vi "PMT-lock-in ROTATION -single rotation-withplot.vi"(0 "Time":dbl=2000.0, 1 "start":dbl=-0.2, 4 "stop":dbl=0.4, 5 "error in":errorcluster, 6 "Frequency (Hz)":dbl=2000.0, 7 "velocity (mm/s)":dbl=0.01, 11 "APD counter source":tag="/Dev1/PFI0", 12 "Interval (ms)":dbl=100.0) -> (19 "error out":errorcluster)   [LabVIEW 2010]
uses:
  <vilib>/DAQmx/read.llb/DAQmx Read (Counter 1D U32 1Chan NSamp).vi
  <vilib>/DAQmx/read.llb/DAQmx Read (Analog 1D DBL NChan 1Samp).vi
  <vilib>/DAQmx/create/channels.llb/DAQmx Create Channel (AI-Voltage-Basic).vi
  <vilib>/DAQmx/configure/timing.llb/DAQmx Timing (Sample Clock).vi
  <vilib>/DAQmx/create/channels.llb/DAQmx Create Channel (CI-Semi Period).vi
  <vilib>/DAQmx/configure/timing.llb/DAQmx Timing (Implicit).vi
  <vilib>/daqmx/miscellaneous.llb/DAQmx Fill In Error Info.vi
  <vilib>/Utility/file.llb/Write To Spreadsheet File (DBL).vi
  Program Files/National Instruments/LabVIEW 2010/resource/objmgr/daqmx.rc
  <userlib>/Newport ESP301/Newport ESP301.lvlib
  <vilib>/Analysis/NI_AALBase.lvlib
panel:
  out "Numeric":dbl
  out "XY Graph 4":cluster{dbl[], dbl[]}(graph)
  in  "Interval":dbl
  in  "Stop":dbl
  in  "Start":dbl
  in  "MG17Motor":refnum<k7>(container)
  out "Y":cdb[](array[numeric])
  out "lock-in":cdb[](array[numeric])
  in  "Photodiode lock-in":tag="Dev1/ai1:2"
  out "Lock-in ave":cdb[](array[numeric])=[1575.618405636581-1354.780267530867i, 2376.9087046503932-757.7461705623398i, 430.26344393445436-2001.7808909348576i, 274.00880357824946-3233.9431935405287i, 888.5075748796727-579.8898083376234i, -1288.5272699325-2538.9581308616175i, 1814.519128631189-3653.715758651259i, 2580.0434389062198-2021.0268672269435i, -866.6428201396346+76.21564286365829i, 1521.4600711033984-2572.1678721325943i, -595.4162527325557-2083.0235307435746i, -2213.651439951863-2304.726379582989i, -1581.3102291517034-3444.508965588943i, 2963.698823411756-3466.251761677201i, 481.31874465992325-2590.4156650248883i, 1077.5453470367086-2271.1674251376476i, 198.06969556939967-3519.1421862721854i, 2126.002010792124-1554.2537826475386i, 1951.9736792597407-5745.697506603049i, -1202.1061809811476-5047.9372242667605i, -1253.5217513533728-1443.9298926030515i, -2137.041153840351-4836.853717701188i, 2212.4903951925257-1208.6810705385744i, 1183.0549708527803-3817.098140391271i, 2431.6697161632046-2314.138255588717i, -502.1017800179644-3590.6658275236773i, 1823.0672697368907-2486.578868433814i, 325.79092146215373-3610.284263297886i, 569.0882415193973-1599.4282971963353i, 3604.4445594698154-4299.084099003819i, -1486.317634221812-3764.9834009605543i, -936.0268941833114-1644.1672785866663i, 292.4719293881775-2213.542158236794i, 318.9126890705529-3399.5505121690685i, 2176.4211819849957-1734.6139938020951i, -953.3489073228936-1819.9444385577192i, 2588.5498347626085-1667.03179470835i, -1029.7581374768777-4091.2934217259995i, 2021.0392661929118-2696.896974507213i, 1446.7594755721875-3062.0656501211965i, 896.0183055508568-3577.8143635934734i, 500.62347573888036-4189.918427475723i, 110.42931799715957-3202.0014798287652i, 1380.892527892701-31.67874295288169i, 2004.357779053466-3723.2441111391868i, 1533.3345211084109-5425.565755113332i, 4364.135929502945-2877.434664532994i, 1257.8199986491823-5604.62816893496i, 1255.4653962401853-3212.376740460875i, 1308.1516341284914-1771.8716117456422i, 5153.052050385331-2811.678589495896i, 1355.9361808963736-3679.095640287204i, 2468.122406976211-64.5200597946781i, -191.8770322387612-3987.068653237768i, 2216.7815087525064-3974.7865562586812i, 811.1736358070949-2695.2342284855467i, 2799.6354672167445-377.1654452867725i, 1232.1759963228278-2564.1871307341107i, -612.1595688464043-795.2702470245148i, 1491.1312054147534-2415.392098859457i, 2503.052266186264-2070.3324822117393i, 1232.7885043542053-4349.227949033147i, 2198.166504463149-3917.0252303013986i, 3670.498177889123-4750.584371253087i, 1049.7577709417797-4272.772555595173i, 5219.707004524125-1875.1488939589096i, 1775.370073504267-1636.5169106622857i, 182.0049681671236-4800.672748236866i, 1484.4660201569386-2355.873769649259i, 1180.3743379538816-3096.2588923411595i, 772.839482950376-1303.4236258336866i, 1549.9878546671623-6153.910783877218i, 47.914672339113324-2471.481982105196i, -2996.873617434996-4030.907310697404i, 2179.4047715196602-2190.9435841994223i, -1253.917311902031-4251.133411229375i, -666.0664524021325-2716.4388438333253i, 2366.5511527892622-4388.085109381615i, 1144.487614423424-3108.4279901249i, 3215.2297186251376-3286.077498973359i, -2099.4212370216474-3992.9683286935906i, 821.6004184060433-3180.0929231557093i, 505.29024588883806-1175.490759941422i, 459.6869492084121-5440.359151670178i, 897.1741551100467-2797.6567465972225i, -715.251854275629-4444.1499126874505i, -392.6708280128788-4277.723316797537i, 1818.1920888630784-2260.469810578464i, 2820.4585961324674-3295.0628100957574i, 901.7716895731513-3808.91683958497i, 2197.026105691963-1790.338710230202i, 3516.3398245212875-4396.432964245725i, 3140.9683427347954-3560.206476639805i, -297.4601035595252-6652.839678247998i, 2423.649156341772-3610.5951839245477i, -669.3988195260619-5549.785379880692i, 2140.7327741099975-1863.2281007983468i, 1183.481250478131-5805.0618816517135i, 649.705046261852-4561.171961145662i, 536.6278860470271-6367.077600133586i, 2950.853999097596-4102.535083107555i, 2600.519648862765-2214.5762658985313i, 2377.7508979599465-5388.334575899893i, 1808.695648329345-4369.762899527957i, -1374.0277904112904-1593.153029070302i, 1091.7884376939294-1260.670032252601i, 304.1154584761832-5567.168439100472i, -981.4392899572041-5080.2068823010795i, 2334.8207050837145-5195.204705625067i, 1026.0461525520295-2069.3530721213815i, 2451.6963287267326-5204.362144252449i, -457.07442892523954-4530.848217232627i, 1448.4675260975769-3703.542478400782i, -139.3301300114125-6171.845273134681i, -638.5494225411103-3042.7814299211786i, 836.4493886595066-5194.499239015591i, 4083.2545653137086-3715.3991686367217i, 2810.0108324746325-2942.6225697417813i, 759.4212715648375-2377.1759813419703i, 2381.5026388043298-5282.685521239267i, 3842.3491663279096-3538.1939118229166i, 4107.981184439802-4482.028922780051i, 4188.535704530702-4431.638680818972i, 2622.805061687113-3225.044270443636i, 2320.0408164989244-5506.118437667573i, 4733.871150582911-6726.079493601502i, 1215.8496144855626-2012.8662115061009i, -533.2529951016124-3411.0893784284817i, 3644.173088205299-3633.0667675324107i, 3270.672994482886-3873.4145432672726i, 2111.2936695423305-3534.34925451735i, 2154.2353903099734-2399.833843699712i, 5054.243227569061-2753.803721852707i, -56.45164399137748-4038.4049421212617i, 1478.965032062944-8093.284127952804i, 2387.809869177338-3421.6143761555795i, 905.8600180472704-4280.089794207029i, 1167.9761571101933-4807.61154339191i, 2615.006809102998-5061.344202856609i, 5736.0218405457545-7406.057718262208i, 2087.149131407617-1955.3279233788548i, 948.4800480918925-4594.139729285302i, 3139.012629546095-6765.397296171153i, 1420.470992347951-5382.169689346777i, 3445.7663547749776-4544.194313423124i, 3201.513005693168-2941.5999006229986i, 3049.9336370159685-1158.007902042452i, 2861.5908669288833-5042.927937990892i, 3095.9352635655273-9215.194383301981i, 2039.8615756080867-3732.315434450052i, 1403.8112843594183-1596.2751532830828i, 2545.8562757136283-5314.4090804453945i, 1215.3340538700709-2860.4819306523045i, 511.8716581082042-6949.692527491928i, 1809.8402634609465-4170.701581866224i, 1983.4607774157303-6035.908248310845i, 2752.5388621309908-6089.687105796719i, 369.47893038169406-5111.808157222528i, 3094.2046544310415-6055.085104732612i, 393.2964691176897-6516.055517047396i, 2888.0442175269045-7598.7063277771795i, 2031.1829482164803-4507.499609177696i, 1286.689454116021-6167.992540949457i, 5898.792902286471-6307.398221312562i, -752.3240471967462-7036.154374283361i, 661.7732013776628-9053.440012958048i, 1343.9313451110952-7300.1365150680385i, 1409.2166078499054-4353.6006586350695i, 1319.979807062355-6098.946164044407i, 2650.6676320636348-6713.891596934963i, 674.1552177359422-5915.62441705174i, 3774.0240383235837-6240.564229457563i, 2442.2611560948644-6293.2324371160375i, 3195.663634320999-6960.896051196942i, -1440.7125037445865-5874.2812237151875i, 2556.676353026318-2669.1223205575393i, -177.91447697888032-4420.9979098207i, 918.2672041740103-2696.085793660552i, 266.11624646743354-7089.299508598139i, 465.92571257727855-3112.388597098675i, 2682.0623447087337-7824.876084863631i, 4426.760086777614-7163.480624926065i, 72.418199475638-5525.248134633922i, 2840.4684511518744-4430.394194406008i, 2819.18026213846-4090.997860405245i, 3891.8677914991113-5735.681669839178i, 2582.946348733788-6972.788033682008i, 4396.446981258371-5272.910199984774i, 2527.0694028279963-7180.483205691042i, 2005.8355590023666-5022.379414766889i, 4150.5132191837665-7929.531405210346i, 1302.0321986691608-6354.158853952622i, 3276.071312110827-7137.673634990922i, 4112.351344872533-6809.4887694552235i, 3233.240880674217-5713.885210511878i, 2294.125519119039-7149.913211378586i, 2521.825788957482-5327.505448819114i, 4472.642628671886-6719.528858266076i, 1156.570051540259-6042.931068163441i, 4263.312379237701-7354.80045290692i, 3231.5904372730024-8603.646792538973i, 2954.9382594092604-10493.056880345923i, 1386.493795027244-4351.668054824362i, 3225.5987563761487-7125.386281538512i, 2998.2482884144883-8640.063883320861i, 5034.563279599767-6334.290206381059i, 5415.675544216023-7053.302845855882i, 5696.215560860752-4634.538974053647i, 3641.080159251063-6410.635909506378i, 3047.4325898702286-6570.782759795123i, 3335.9774335594325-7959.350599243415i, 1034.8217959811998-9471.783462254887i, 4472.18270995681-7972.728001848677i, 1687.1669694183852-7691.372201957279i, 3838.7682454706164-4608.7353483079205i, 2789.723450221373-6735.727257013259i, -100.86652927079496-8280.414793254728i, 2691.163672840396-8195.965205608558i, 3135.3844380749388-4334.554385434998i, 4754.501592156671-8150.319779417582i, 3152.46020482383-5267.56497828292i, 3345.6422634325527-7666.082415105115i, 4268.253179283182-6228.07112408391i, 2468.284969279949-7082.494872178709i, 5146.391606558882-9442.984964408635i, 3017.350279911123-6366.988520079154i, 2983.935453577272-8328.674529063186i, 1779.3304772234042-5359.456608012244i, 3510.110664729989-7196.888677953726i, 2937.7827141235925-7916.234771289581i, 3390.6936769238473-6158.017390219011i, 5116.173881936087-8156.452921998013i, 4815.733340806664-7292.728942666812i, 4745.333271691776-8481.200756112174i, 5365.885743637579-4990.0099400448125i, 4782.323630181974-8164.634702569512i, 3551.0138437730548-10338.68778651241i, 4487.380002158204-8108.007387676075i, 3286.690337470376-7921.318236867741i, 3376.0031275370734-7442.806636330388i, 2265.3725204363504-8070.769839902126i, 807.157044198946-8219.94254152485i, 2523.9981278773407-7171.667112435127i, 3364.1321813453346-7864.664176825664i, 2853.3817229355914-9339.871887243396i, 6505.60918603455-8014.805912068681i, 4548.785193789941-7068.753744337186i, 6491.907317829052-11153.440489008437i, 4119.273108721625-11156.272587046135i, 4468.012071037022-7603.962904432309i, 2445.5704319838724-6135.840418565561i, 5415.917334042106-7934.862125438665i, 4375.69619385447-10252.680472604265i, 3300.624533464226-8981.870565534917i, 6416.737775940689-8055.459849998011i, 2147.0423638877305-7800.421166609077i, 3470.9244469034734-9652.502973243401i, 3834.944754020379-8997.730145163221i, 5191.853577022501-7983.604511323078i, 6926.471309680483-9982.320605300636i, 5565.609902585673-8801.550363525452i, 4425.618931406877-9686.465846148525i, 4750.691251487348-7229.1346402430445i, 6060.328452057632-8410.696096223492i, 8642.740346806098-10615.813484936069i, 4000.851811107144-7713.603497846788i, 5340.429627507394-5564.470385899507i, 4246.436081468988-8451.254786399202i, 5142.1808707504315-8970.507919104013i, 5849.381578431081-10722.75061539895i, 4743.6306751765815-10982.737699019313i, 3662.8719327485355-9718.164212385662i, 6375.327301060715-12608.26617199092i, 3208.3276860287815-13184.554856913566i, 6462.5111596734905-13846.584482642662i, 6450.4053011412-13032.71550445879i, 6611.623790823844-12964.883545718125i, 3012.9070584814795-12009.812713614641i, 8276.19374857804-9520.97744420273i, 6088.451995458484-12662.88351339309i, 7433.678429940602-12919.825710196095i, 2852.2427242612903-12793.526883177705i, 4723.55739094081-11279.148288208788i, 3539.2212584925037-12636.463067970388i, 3127.94039402949-13919.258461339436i, 4042.7498170819094-10438.47267823518i, 3313.8462354475123-10185.0005143772i, 2083.0105152702654-13337.796688349425i, 4415.742453714986-12296.444745051213i, 2333.6873585833296-12599.213531007452i, 6541.907912842064-16769.193637528468i, 3868.710658608924-12774.742387506203i, 3516.06243618668-13159.889412777684i, 3703.0889476515376-13765.671181982048i, 3675.6227579825686-14310.612784302477i, 3812.441605180332-10887.472287294133i, 1397.0828808435276-13734.236307413365i, 3938.7295726058055-14035.867119071843i, 1825.260919517559-15010.104724879697i, 3484.4101933582256-13615.583679334506i, 6045.007586638047-14483.223663464456i, 2266.133309683563-12932.45957066616i, 1216.366596052904-12096.177750738301i, 3094.775105021804-13466.285271132703i, 1343.0682931154638-15830.12324274869i, 3723.6282011488-12088.74110571i, 527.3450422106561-14712.257687544445i, 3319.7368165379435-11364.549104548822i, 2297.976854474832-14017.971969481849i, 848.5790411140356-13690.064307972925i, 2033.8439056264206-11773.725311700986i, 770.4447513128919-15217.642846257875i, 1853.0905652266492-14177.448493715083i, 1792.8092173986097-14424.43565501314i, 1207.0272513039884-11125.9188243898i, 984.5665559117601-10123.787770201357i, 1934.1627600043782-13763.568829080928i, 3319.8803814773346-12100.916557943508i, -682.4754463650166-12295.072338224982i, 1010.1082259658396-12544.228333526644i, 1443.8085907844304-8732.055376323178i, 822.8876816006555-9900.247376109055i, 1611.2724688688406-10996.094241351546i, 1446.180298133071-9565.616335014467i, 939.6520132331581-10622.586263289028i, 642.985545092809-14054.122868742952i, -1312.8387064380534-7879.215014987034i, -422.0499978802597-8294.918016716652i, 945.0198134398789-8873.172496645318i, -1874.029242704319-7324.3221632276i, -911.5088864967161-6727.6651678308735i, -814.0487519371331-7309.334312834168i, -8.383164099631617-7717.6915717605325i, 1244.481834156355-6580.924107883921i, 2358.0710913512617-5494.890411171763i, 715.2405105254029-4605.4887026423075i, -1350.4053391373088-6162.0264940668i, 840.2512985319834-4720.024981664563i, 244.63112371075078-5910.131730889196i, -503.3729172442221-4348.932318470168i, 815.7115745334273-4384.529220903181i, -443.19112139589043-4965.184510612029i, 210.21261276302315-3120.9557463527262i, -1835.4249558866986-2538.6010144168818i, -1123.917602737967-3779.9767572298338i, 660.1740596516721-1772.286398958819i, 1102.1856160660475-964.6607531448776i, -733.3571432042307-5349.184027686582i, 839.6615019045682-3137.2615174093594i, -1871.8261810359465-1294.6855534867075i, 1531.2808862634479-1171.163074759485i, 667.9924422761186-2953.8871853082583i, 129.02940560864587-189.19271316344606i, 3182.1888736477886-2735.789162005561i, 1168.9250333431555-272.33635084978556i, -1123.7362237647644-3604.17838791847i, -1395.1851983393085-1895.665289942973i, -571.7555591978203+1071.1038162245345i, -2170.2022145503834-3487.684684038925i, -776.6818955944391-480.1729930056903i, -1854.886019995663-800.1289791333481i, -1176.1015445632427-1424.3339818833902i, 1687.3748265199076-2187.0524559081196i]
  out "Signal ave":cdb[](array[numeric])=[19973.709551616634+2137.68316236515i, 17641.679526528722-590.6971995647476i, 18964.42920598725+784.4848963807648i, 20443.339940618058-1292.7777293085899i, 18783.5054836337-586.7016703281453i, 17591.273408972083+346.8128608267923i, 14435.708762127228+355.6367697407369i, 17955.809692629875+970.7427647798825i, 18901.743132287455+2350.1528064430026i, 16181.835360198562+769.9403678944353i, 18619.57566660758+101.29369171834527i, 19714.78151159957+2874.616325663279i, 19910.019889764048+1971.0987272756875i, 18778.497214983232+2012.7224915615561i, 19243.150553663443-879.2727034505004i, 18798.14167792132+939.01546450782i, 22779.513628065473+2910.1695280022336i, 21017.14310563447+1146.5352790872914i, 22370.876093470342+3759.021856982118i, 22038.151641544195+2119.3106285164895i, 20021.386988714767+1152.1162632125843i, 21872.217528511355+2454.1895448417736i, 21877.851134885925-117.33523182960502i, 21685.988414070882+4080.139956736632i, 21687.794636398055+4650.407322525038i, 23216.427067114826+365.3502429257846i, 18649.66991238834+3200.034227192907i, 20283.547667981533+121.5380892072013i, 21996.53785526474+1247.1035231835428i, 23187.751052088097+1585.2474258033446i, 25751.290144574323+768.5946057235767i, 23093.45018600484+2197.702088670342i, 21645.07391481427-149.9515993110738i, 17628.63439529744+3672.495048304777i, 19950.242163716157+2209.1177096797396i, 20492.098732128667+1793.4072912054614i, 19449.224016281816+3379.3313636089556i, 20175.360044553425+3508.299044497772i, 21079.557314354697+1546.639742437651i, 22785.549397207353-591.3827688982097i, 22077.17826531066+3270.940314774405i, 23398.14028789829+2830.2652332386506i, 20646.262168996647-126.72623217786679i, 22349.320346499582-31.902379363178866i, 24243.400587859025+3426.5148490693373i, 21916.085290303516+2529.5297370956946i, 21981.748030513918+1530.0184869116495i, 22220.24447104533+2731.5080444137875i, 22945.91165334838+1386.5913250565343i, 22707.88746616709+959.3818222670607i, 20273.53720619981-63.13732196241676i, 22042.231102113492-19.60268674334982i, 25650.121706604354-1289.452205628714i, 22690.294811693293+1628.8665056493544i, 23952.7408549437+1505.7600996787273i, 22845.286418081443+855.7065280668362i, 24593.853888002035-55.12625244238829i, 25077.041608896685+1491.9633380572377i, 25068.358254862625+1317.2389077564858i, 23548.43171700486+1611.2100374579366i, 25969.705099151113+388.3654069151239i, 23702.173502861428+2015.8803757325109i, 25965.49633041593+2170.8831987562753i, 26701.80741871982+278.2637036757209i, 26860.199652986015-3275.5802176156444i, 26488.641761538747+1822.8973333641702i, 24914.763925257383-1756.5451070743327i, 24540.892320736584+2643.699533046424i, 26346.68660390194+2976.8179266998004i, 23236.44710958339-456.99626328409965i, 25552.947774671287+2296.2714910902637i, 24809.85032506418+3461.188281980759i, 27374.123718323208+2344.9869732905986i, 26281.683954696782+3069.656547340776i, 26683.785078787205+713.8589978246326i, 27018.240909618165+1228.2539625246457i, 26299.67568231255+2257.2555548593223i, 24921.943873921533+3476.991048682698i, 27963.693598569236+2024.1104863223575i, 25338.366480063796+1460.8181084882951i, 29096.956578838577+2852.7644971285185i, 29099.59494568991+2708.1173513220506i, 27156.515231099107+1477.3327428415637i, 27621.35094330793+254.29043438568937i, 25450.491878025037+2740.910850675434i, 26928.105928600937+309.4305324651831i, 27887.833450880145+245.37632737638654i, 25628.298853828666-991.6321417652896i, 29018.592445695496+4265.022956712465i, 27655.547923423754+3309.082973772353i, 27654.10848220132+503.6750065510531i, 28091.70288293553+3312.482883066248i, 28857.703507639355+2717.4979820902295i, 29239.16353925298+846.9422025653236i, 27633.945284273672+950.8074087747111i, 30817.8953983305+183.09505881489707i, 28716.053737316877+1359.63211416521i, 31368.296864577864+1285.0617682950906i, 30394.766926577733-64.2060995609443i, 30639.02392489712+1903.0823876456561i, 29889.982496973058+1288.5353310469095i, 30092.068332835745+2556.940302097282i, 28447.660023560045+131.4721229425815i, 33747.72123923668+2604.592206852926i, 30733.81223686092+1711.5814227720543i, 32109.547759341844+1571.950999302157i, 32242.31561562917+1393.6930049698697i, 32590.39968579184+994.9027982538349i, 30826.777950969077+4965.444045031032i, 32436.07511683829-508.22337870489105i, 31859.064193175956+335.5035319454363i, 30734.76537878668+2275.0504484911216i, 31616.526804989484+1156.3420961595307i, 31726.168231515585+2058.313894580561i, 34072.22274345362+1727.996383661928i, 30735.246560596046+607.2659759455697i, 32722.61019328942-304.4169498497065i, 33379.36582025203+1398.4899414019935i, 31283.35823156214+2067.1972169709866i, 34276.5412407718+1801.202047655149i, 32524.364278892383+411.72304514708674i, 32911.84465016063+3106.4363661109296i, 34144.52154366048-674.2921396242247i, 32213.46494533557+1497.193235188105i, 33359.57364425402+4890.421863521732i, 33020.841577154395+2432.091933361664i, 34645.64981776737+992.224198121691i, 34935.86915287571+3139.85366888939i, 34053.63229435785+1902.4338552972958i, 35190.1445344589+3684.5700980275315i, 33810.07920022588+1946.6764540660133i, 37192.40763536752+2291.5382514440716i, 34390.850778472406+3552.7818186234745i, 36523.90485411221+3552.3812997237105i, 35928.96030095971+1527.1878693068945i, 35101.623255081235-422.12491807187314i, 35874.32004068537+3995.9013181685286i, 38245.00604558553+2794.963564772352i, 36282.57405831285+2289.9622033544665i, 35801.267580883265+4612.021916772325i, 37913.50698705951+1810.1753523431848i, 37868.538496427704+1191.0366636643264i, 35433.08521708961+3281.138887103279i, 39933.430938674246+907.6894155147743i, 37197.9365283357+473.98998197129714i, 36551.44941131433+334.6769403013012i, 37718.6079672964+405.8678874777269i, 35936.98611716157+3673.2883676638235i, 37899.705096743186+4498.070132155895i, 39012.34346929452+3905.593779920433i, 38502.32920850229+2135.9721312509164i, 40447.2529957549+1518.378412117692i, 40209.58476152285+3464.9226117868006i, 39179.87322920747+4498.566856320326i, 40135.85181622762+1967.805904084847i, 39633.94042233719+4445.4072774265205i, 41424.06052762676+2912.18379277977i, 40531.01365901944+3373.1736448150123i, 38643.12888467001+4193.790711494204i, 39027.153852419324+2248.685628882114i, 44654.11961569351+952.1317955274311i, 39944.82064738734+1383.9756797142338i, 42636.26359705652+1343.2573124938638i, 43028.84813983183+3538.8834076296994i, 40359.93711784901+4334.420837491159i, 38658.037995574734+2261.4151424959105i, 38420.68131891876+1264.5325731248104i, 43911.426293769684+747.554605029913i, 38009.551880513834+3552.0732622099863i, 44022.31679663538+2495.6957059671213i, 44496.056984881165+1604.7394074286194i, 43178.600994714994+2885.0449554090123i, 44198.01437631617+502.34729455858894i, 42764.84151033523+3212.966631358569i, 42592.107908395585+1668.6815654216025i, 46034.78812228002+4455.730401066182i, 46580.98252889817+3778.266571802271i, 42050.55243452278+3758.9881368248584i, 48205.45224925414+3462.2732552830926i, 45118.651222056615+2929.6518139001864i, 46956.83137800294+3894.477330360894i, 45501.89150707532+410.8961765597546i, 47780.722456232+3260.665707046737i, 44659.73126251827+3019.103741251046i, 46104.95132677405+2834.695923843316i, 47438.76549627922+3901.244860974728i, 47574.23814215162+2564.47225164935i, 47333.77920621191+4833.004044079297i, 48674.36715884112+898.7979723580138i, 47913.71587388793+5753.460649058702i, 46680.79468934667+1828.8276025492314i, 48747.78242159783+3830.9906332830196i, 49493.82194100686-1147.7435192922012i, 49238.97020889669+1217.3806166213337i, 49659.41497869748+2896.0220275089414i, 49922.467736578175+976.3014341831184i, 48122.218330009746+4044.246307736089i, 50728.933260013655+2301.9555702623406i, 50426.48650279836+2622.593932015488i, 53111.54386920386+2592.047770207518i, 50379.18284070535+3996.648332231636i, 50833.74129682521+3827.5323787287493i, 50276.528475600244-397.24418561847347i, 52521.73784220521+1215.93732991796i, 50727.59448501055+1587.0299271466995i, 52774.08272609958+3168.678810043082i, 53530.35354307037+3153.616420441528i, 49400.85628930751+2483.4779682878993i, 54576.30053668804+4515.088010859563i, 53210.843520241506+3485.18810442704i, 54808.731176971865+2805.6714446276737i, 54131.65617607714+4708.274692447471i, 52050.97491552243+860.6104775218644i, 53846.03228996166+3144.825781282068i, 56437.45630070019+3781.521907374692i, 56872.44923672083+4740.357738623805i, 56506.976569706574+3571.6972230511424i, 56122.1625694851+5064.461210812666i, 55552.439949603744+3217.5911785784383i, 54197.08525324574+3065.799700794284i, 55351.29814379563+5277.107333139463i, 57022.28910243668+2020.5423545949095i, 57966.34735640804+3790.530471207716i, 59215.871189722464+5746.952903378195i, 55853.27951363862+3370.432688647369i, 57971.10026426304+3902.920247338582i, 55575.962320089995+3946.349866444711i, 53919.41630411781+4190.446809659357i, 55992.59602380357+2597.1179953191076i, 58925.31937109892+1881.3178312811253i, 55152.48768021333+4823.910074913119i, 61550.851147975074+2923.6268947041003i, 58025.31157427309+4423.737991353994i, 59953.05368253878+2628.9658176630023i, 56731.86829871749+2344.614900096433i, 58329.518773108626+4631.775781435258i, 61422.440267130434+2258.5760540698116i, 62045.67950061424+542.0322484292351i, 58957.44508030157+2376.8826163311924i, 59829.80588693156+4530.9213058834985i, 60115.67891516981+7080.701980317283i, 60865.784617930076-392.0492100132247i, 61520.315840997515+1346.916327792884i, 62669.975399233976+920.6776954421268i, 62599.45803377901+4176.317544211401i, 64096.245997110505+4132.454017068202i, 64924.98977651045+3982.623708867158i, 67352.74184301558+3867.9328257361894i, 65408.89287634846+3280.8053428012463i, 64561.08345370794+3457.3649032173084i, 67933.9733797803+4312.1263237779i, 64997.73200022106+5700.128391838776i, 65178.453628589734+5928.007376987131i, 67058.91471038818+4137.3498495279155i, 66422.00948928189+3550.307954967456i, 65439.604361950536+5442.195117047383i, 69707.11726364907+5908.003955378939i, 70501.48114958392+4270.954851555873i, 68099.18287494844+5085.339780590591i, 71207.08603062917+4988.153126414789i, 71305.2745976459+2449.914709389416i, 73299.78008493187+4072.663481611199i, 71198.5333353847+2663.292271019781i, 72747.37634043346+2066.3868712407207i, 72537.35439987564+5332.394637655405i, 72822.80196767036+4717.687067031672i, 74110.37560523134+4070.0717297584083i, 74090.76916031171+3712.8083610513972i, 77532.49749680342+3916.912486215792i, 77855.61000565469+4244.644783549382i, 80141.13389083299+3568.9960639135816i, 80096.29528802745+4478.341703421639i, 78878.80665780169+5271.018286940097i, 80834.22339497734+6058.2314951689605i, 82551.58375247684+2968.2393827156966i, 79961.11900757885+4036.8180392654126i, 85322.05433041895+4375.581534713559i, 85674.32244881566+4120.994111269414i, 85814.23398049959+2778.1549316530813i, 87229.4987262963+3301.127968348004i, 89089.2304542043+6634.044264508146i, 90207.16067887297+5700.129391349136i, 92896.56488139722+3753.9567239860407i, 93358.11169050074+5741.308700361177i, 92862.62270723494+7308.441357457153i, 94044.8749091163+5317.911739504252i, 97206.05897811196+7493.372092573997i, 95203.60075421458+6466.563427418022i, 96635.2218642239+6360.661086563576i, 99223.00304946786+5944.922717782365i, 99604.33261943738+8341.485217075271i, 99205.87135539162+4700.30084507866i, 99636.59329708801+5280.88441507546i, 100305.18791388128+7899.87619089107i, 102050.84518525499+7039.313760840313i, 101963.09211888627+4196.707865676357i, 104815.58839322721+4291.404572448898i, 106007.31466316282+6235.22732367124i, 106609.44430278087+5759.485308884078i, 103894.51820826704+6253.566531548679i, 104537.244768498+4935.355572246167i, 104494.31290463262+9238.708466288446i, 104556.61686128186+7305.011221231405i, 103116.14370030162+8340.001515539703i, 101531.33165206132+6108.114347233464i, 104220.65301927809+8029.629028542398i, 102930.77897828724+6102.658516566913i, 102006.32555247868+6686.477306991325i, 101456.17809984833+7585.061130233768i, 101487.76699549012+9933.727119501966i, 99739.96200283422+7162.085932781197i, 96871.99872036949+6277.45473389155i, 98567.49091580088+7496.920314989954i, 96082.9326907551+5292.609874919571i, 92739.44655875764+4948.650055115154i, 91871.171097579+8349.247350111758i, 91843.8898712052+6009.600483014275i, 89160.6478151269+4589.728818531861i, 85472.86835798915+7151.307495948784i, 84104.77649438687+5867.1315478274355i, 79616.0107260644+5228.576623307221i, 79376.79332933357+4765.336420485306i, 77702.25305853519+5232.4582736282355i, 72701.48417190262+6588.268568987635i, 73532.31207469966+4994.50278815127i, 70307.39874848313+5186.401005366064i, 67062.89234606267+5481.48035032536i, 64557.99582654852+4906.663328007538i, 60875.701734046124+2706.9587995243883i, 60426.95915963755+4948.609671342333i, 59440.477733183165+8582.2965618034i, 55123.16184466921+5916.508027120281i, 51274.635170264904+1410.0599732277517i, 49958.61413848713+3754.093398380502i, 44624.80379097324+3065.0079653166945i, 45741.14874078798+990.9722777927909i, 44603.42578545316+5402.720264030694i, 40581.08221931923+5176.026308233984i, 39789.43314494175+3404.63470360218i, 39449.453501254146+1280.9785138570319i, 32793.564450075624+1020.6869533548776i, 34591.37422849459+2762.3556005513638i, 30996.585395681734+1768.194873735904i, 29612.862259743142+1184.5433813177294i, 27388.35780925263+2188.9682093427946i, 25524.19384460949+1919.108800077599i, 22531.903920834222+4208.8895354181195i, 18782.612144186307+567.7782084369536i, 22514.091544228137+1573.8895677931453i, 17751.56036733101+844.6024127716448i, 16051.48666175705+619.0264003980495i, 14165.122611183091+2333.9407596662877i, 14236.673827335766+1688.7368700689615i, 12740.750110461735-75.44163707900623i, 11060.153931690775+2663.6027877716915i, 10588.82496008224-152.32858361143397i, 9927.00591358419+2010.254229709676i, 10769.007589051082+531.6279166855886i, 9089.419983528307+1187.9772418695518i, 7245.387153267173-1244.554893578811i, 5758.050689958366+2526.1594470154505i, 8520.419910027122-975.9717690913108i, 7602.600382534072-521.1368712546655i]
  out "Position":dbl[](array[numeric])=[-0.0006666666666665932, 0.00200000000000015, 0.018000000000000054, 0.028000000000000063, 0.03733333333333348, 0.04666666666666671, 0.05466666666666675, 0.06466666666666676, 0.07600000000000015, 0.08333333333333341, 0.09533333333333338, 0.10533333333333339, 0.11599999999999999, 0.12466666666666681, 0.136, 0.14533333333333343, 0.15666666666666682, 0.16533333333333344, 0.17666666666666683, 0.18600000000000005, 0.19866666666666682, 0.20666666666666667, 0.21866666666666684, 0.22800000000000006, 0.23866666666666667, 0.24866666666666667, 0.2580000000000001, 0.2686666666666667, 0.27866666666666673, 0.2900000000000001, 0.2993333333333335, 0.31133333333333346, 0.31933333333333336, 0.3313333333333335, 0.34066666666666673, 0.35066666666666674, 0.3620000000000001, 0.37133333333333335, 0.3826666666666667, 0.3920000000000001, 0.4033333333333333, 0.41200000000000014, 0.42333333333333334, 0.43333333333333335, 0.44266666666666676, 0.4546666666666668, 0.4640000000000002, 0.4746666666666668, 0.4846666666666668, 0.4946666666666668, 0.5053333333333334, 0.5160000000000001, 0.5253333333333334, 0.5360000000000001, 0.5466666666666669, 0.5573333333333335, 0.5666666666666668, 0.5760000000000001, 0.5873333333333335, 0.5980000000000001, 0.6073333333333335, 0.6186666666666667, 0.6286666666666667, 0.6413333333333334, 0.6473333333333334, 0.6613333333333334, 0.6673333333333334, 0.68, 0.6906666666666668, 0.7000000000000001, 0.7106666666666668, 0.7213333333333334, 0.7313333333333334, 0.7406666666666667, 0.7520000000000001, 0.7653333333333334, 0.7693333333333334, 0.7840000000000001, 0.7926666666666667, 0.8026666666666668, 0.8133333333333335, 0.8240000000000002, 0.8333333333333334, 0.8446666666666668, 0.854, 0.8653333333333335, 0.8746666666666668, 0.8860000000000001, 0.8946666666666668, 0.9046666666666668, 0.9166666666666667, 0.9260000000000002, 0.9366666666666668, 0.9473333333333334, 0.9566666666666668, 0.9666666666666668, 0.9766666666666668, 0.988, 0.9986666666666668, 1.0086666666666668, 1.0193333333333334, 1.0300000000000002, 1.0393333333333334, 1.05, 1.0593333333333335, 1.0693333333333335, 1.082, 1.09, 1.100666666666667, 1.110666666666667, 1.1213333333333335, 1.1300000000000001, 1.1433333333333335, 1.1526666666666667, 1.1620000000000001, 1.1733333333333336, 1.1826666666666668, 1.1933333333333336, 1.2026666666666668, 1.2133333333333336, 1.2246666666666668, 1.2333333333333334, 1.2446666666666668, 1.2560000000000002, 1.2653333333333336, 1.2753333333333337, 1.2846666666666668, 1.2953333333333334, 1.3073333333333335, 1.3160000000000003, 1.3266666666666669, 1.3360000000000003, 1.346666666666667, 1.3573333333333335, 1.366, 1.3773333333333335, 1.3873333333333335, 1.3980000000000001, 1.4073333333333335, 1.4193333333333333, 1.4280000000000002, 1.4393333333333334, 1.4486666666666668, 1.4586666666666668, 1.47, 1.4806666666666668, 1.4906666666666668, 1.5006666666666668, 1.5106666666666668, 1.5206666666666668, 1.5313333333333334, 1.542, 1.552, 1.5626666666666666, 1.5713333333333335, 1.5826666666666667, 1.594, 1.602, 1.614]
  out "signal":cdb[](array[numeric])=[-158.66309241065937+0.0i, -144.7080289226683+0.0i, -193.81938365073574+0.0i, -277.51044014376885+0.0i, -202.28902697601643+0.0i, -167.6555317980792+0.0i, -215.28220591579702+0.0i, -161.15918857602446+0.0i, -233.33336296272773+0.0i, -120.72837078291104+0.0i, -204.57920410294446+0.0i, -87.29007401773652+0.0i, -214.7991892223199+0.0i, -199.65497771760784+0.0i, -239.65628211683907+0.0i, -215.51896289175966+0.0i, -125.8567333947849+0.0i, -159.42195589099265+0.0i, -169.6546538525181+0.0i, -149.55718821232585+0.0i, -154.69524850987636+0.0i, -245.17625377062177+0.0i, -236.82917241850873+0.0i, -255.121218250958+0.0i, -102.23055534800642+0.0i, -140.84225285108232+0.0i, -249.45615968348193+0.0i, -184.05945330462555+0.0i, -153.48797682498116+0.0i, -239.6574322622182+0.0i, -165.50316549974968+0.0i, -215.25191421799855+0.0i, -233.43799668220345+0.0i, -156.7745137030265+0.0i, -191.63735292818+0.0i, -111.97740059311627+0.0i, -181.6706696430092+0.0i, -325.82654010231363+0.0i, -234.3086162061145+0.0i, -174.6569255305385+0.0i, -160.41049694262165+0.0i, -183.31411890419804+0.0i, -165.07626254894285+0.0i, -193.71097650962383+0.0i, -253.9010129354824+0.0i, -149.28532362963142+0.0i, -216.44653245735117+0.0i, -200.51596056734343+0.0i, -185.66227137537726+0.0i, -208.88782542956278+0.0i, -200.62506290752435+0.0i, -224.1360565601526+0.0i, -198.68542270613352+0.0i, -212.04415204083807+0.0i, -184.15000402760234+0.0i, -205.13638758590332+0.0i, -170.1507212058268+0.0i, -190.82301704084148+0.0i, -151.09148108683212+0.0i, -172.77321016491624+0.0i, -217.85033787039447+0.0i, -124.87205403627104+0.0i, -256.8460626993897+0.0i, -169.9716193690474+0.0i, -197.98553107791076+0.0i, -179.01866380364754+0.0i, -211.363698039444+0.0i, -199.34278427179834+0.0i, -189.8776248629215+0.0i, -187.5789908297479+0.0i, -184.6024996450201+0.0i, -238.80854224560107+0.0i, -267.04089176939306+0.0i, -174.33496697972805+0.0i, -174.29834734205815+0.0i, -123.59262075124343+0.0i, -181.42537071133074+0.0i, -167.12049899929343+0.0i, -191.39215074239974+0.0i, -206.8176918568056+0.0i, -150.22049402256016+0.0i, -178.55439976468733+0.0i, -217.09043550222032+0.0i, -154.13454253612144+0.0i, -180.7740888518747+0.0i, -218.95425533539265+0.0i, -153.58253399869045+0.0i, -214.48377043506343+0.0i, -175.07896833274845+0.0i, -193.28225126155803+0.0i, -210.02874424372203+0.0i, -209.42921114990622+0.0i, -182.35399586825315+0.0i, -226.72190849302797+0.0i, -152.4087276853329+0.0i, -197.31451459762593+0.0i, -241.28553538384267+0.0i, -184.9648188303122+0.0i, -193.7635813050465+0.0i, -226.7165657410983+0.0i, -175.33323088903808+0.0i, -244.11675745656066+0.0i, -228.93705275356479+0.0i, -192.92572686619496+0.0i, -234.23954677317442+0.0i, -236.28847925218133+0.0i, -184.52290858853075+0.0i, -214.7006409236701+0.0i, -170.04541017553038+0.0i, -207.44662977598546+0.0i, -234.27462858163153+0.0i, -227.33780369953183+0.0i, -186.4839965294409+0.0i, -272.75466673299843+0.0i, -260.0387868378957+0.0i, -188.7063550805483+0.0i, -164.38333160398997+0.0i, -130.74764855471312+0.0i, -191.97639530473225+0.0i, -174.18329189306132+0.0i, -215.6094643242277+0.0i, -184.1062518750732+0.0i, -226.2007033712298+0.0i, -128.21244881524262+0.0i, -222.2483814014431+0.0i, -218.87365766475887+0.0i, -216.58495232429414+0.0i, -160.07516087101612+0.0i, -230.8319572349087+0.0i, -226.34709028489215+0.0i, -210.6884122350557+0.0i, -240.63130186021+0.0i, -217.7916467317118+0.0i, -210.38145661017825+0.0i, -256.6858907566666+0.0i, -268.5203388918835+0.0i, -164.25255985739386+0.0i, -201.44049515240476+0.0i, -182.5167309368544+0.0i, -189.767737423987+0.0i, -176.33049501157348+0.0i, -227.8078269459038+0.0i, -173.29871922880466+0.0i, -229.41615005696804+0.0i, -276.95416992084847+0.0i, -201.49859003164147+0.0i, -189.88090375276124+0.0i, -210.1485224042085+0.0i, -111.10938859197086+0.0i, -277.7038748063842+0.0i, -203.27179344494016+0.0i, -203.5269646876277+0.0i, -166.29596493395138+0.0i, -156.28220421333754+0.0i, -166.1296407472537+0.0i, -215.63190154988752+0.0i, -258.80230667214573+0.0i, -179.72287122648777+0.0i, -156.68184747725172+0.0i]
  out "sum":cdb[](array[numeric])=[6361.729426575248+0.0i, 6300.705036403964+0.0i, 6426.037852404226+0.0i, 6342.805203236037+0.0i, 6396.801745180505+0.0i, 6598.1353322968325+0.0i, 6451.127592449462+0.0i, 6388.9437421175435+0.0i, 6351.233617302004+0.0i, 6235.555318339392+0.0i, 6315.3971790660335+0.0i, 6271.712019154894+0.0i, 6250.116894957981+0.0i, 6444.268453977207+0.0i, 6502.152042715343+0.0i, 6458.870583839391+0.0i, 6259.397880526954+0.0i, 6374.14215539224+0.0i, 6344.344938092168+0.0i, 6305.623023623797+0.0i, 6307.877293397657+0.0i, 6504.69846317249+0.0i, 6458.0830377551665+0.0i, 6502.424968824772+0.0i, 6450.280430659727+0.0i, 6347.839783899084+0.0i, 6267.25071806365+0.0i, 6298.562206372206+0.0i, 6331.05605662548+0.0i, 6331.6713973495+0.0i, 6370.146571909099+0.0i, 6462.70131559019+0.0i, 6308.254954288188+0.0i, 6238.407451259633+0.0i, 6327.197452678803+0.0i, 6317.72704141643+0.0i, 6341.253736850612+0.0i, 6452.563722023134+0.0i, 6529.222341842273+0.0i, 6450.439498947742+0.0i, 6441.44394317778+0.0i, 6283.7440440912305+0.0i, 6307.00046696328+0.0i, 6271.419719577328+0.0i, 6395.960893085852+0.0i, 6504.6349594902285+0.0i, 6599.303405200865+0.0i, 6520.52993558006+0.0i, 6454.3226205025585+0.0i, 6396.869870317343+0.0i, 6425.682429441438+0.0i, 6399.718101447933+0.0i, 6354.931836522339+0.0i, 6345.702012365151+0.0i, 6470.24078702037+0.0i, 6722.664572099743+0.0i, 6478.674411978894+0.0i, 6330.038977140593+0.0i, 6395.831630712768+0.0i, 6427.005644005687+0.0i, 6260.740133282362+0.0i, 6462.904991592876+0.0i, 6475.502436689787+0.0i, 6665.8858685719115+0.0i, 6472.95011960659+0.0i, 6449.204204925966+0.0i, 6362.9716780893195+0.0i, 6375.600140880278+0.0i, 6457.287111097583+0.0i, 6566.745075617779+0.0i, 6607.88629016871+0.0i, 6697.566646983754+0.0i, 6602.742637405303+0.0i, 6447.20082224207+0.0i, 6437.98014285328+0.0i, 6398.476421200368+0.0i, 6321.385470461953+0.0i, 6528.507067404153+0.0i, 6603.018085904494+0.0i, 6669.516943727129+0.0i, 6519.923237164705+0.0i, 6462.496559291243+0.0i, 6482.1128843552115+0.0i, 6320.134562386991+0.0i, 6375.021470398009+0.0i, 6584.27496847791+0.0i, 6635.196504048689+0.0i, 6725.785530959127+0.0i, 6637.369242646962+0.0i, 6517.793971959813+0.0i, 6497.414280403324+0.0i, 6412.499535339432+0.0i, 6366.603372426857+0.0i, 6502.431668917836+0.0i, 6611.89603925715+0.0i, 6647.998803874433+0.0i, 6529.822193737957+0.0i, 6495.925452073076+0.0i, 6354.617446641705+0.0i, 6419.358959756062+0.0i, 6316.09134058991+0.0i, 6445.953186284987+0.0i, 6500.8532622298735+0.0i, 6706.0997917041+0.0i, 6609.141302334519+0.0i, 6577.667047756295+0.0i, 6479.946349985039+0.0i, 6351.3799575574585+0.0i, 6304.852432420911+0.0i, 6365.416714514388+0.0i, 6543.7559352651715+0.0i, 6591.913389610377+0.0i, 6582.217677253006+0.0i, 6532.959155511053+0.0i, 6403.96297636408+0.0i, 6417.573187998254+0.0i, 6404.178852751371+0.0i, 6508.052386709326+0.0i, 6484.934001289769+0.0i, 6585.010224561391+0.0i, 6534.624925670861+0.0i, 6471.5167604295575+0.0i, 6491.235117336318+0.0i, 6406.84686278033+0.0i, 6429.762600828+0.0i, 6545.74947806401+0.0i, 6601.918618159705+0.0i, 6741.117574736849+0.0i, 6490.274351249871+0.0i, 6487.736616469431+0.0i, 6365.3517786945295+0.0i, 6528.098633531032+0.0i, 6400.096883639442+0.0i, 6539.037850451446+0.0i, 6580.677910706791+0.0i, 6696.511386149363+0.0i, 6689.249068585574+0.0i, 6489.338754479212+0.0i, 6453.881319465533+0.0i, 6339.021602760646+0.0i, 6289.507552368182+0.0i, 6418.562939165355+0.0i, 6578.628395039278+0.0i, 6470.395701179163+0.0i, 6606.256913062994+0.0i, 6444.871168535631+0.0i, 6387.05896854104+0.0i, 6250.398901431763+0.0i, 6410.066994577008+0.0i, 6484.67348064254+0.0i, 6548.9575789811+0.0i, 6586.515503291366+0.0i, 6566.354817801783+0.0i, 6451.153032118698+0.0i, 6424.394982368325+0.0i, 6314.021926487543+0.0i, 6285.240226797207+0.0i, 6446.990701650428+0.0i, 6546.3048000460785+0.0i]
  out "modulation":dbl(graph)=-156.68184747725172
  out "sum 2":dbl(graph)=99872.8000000004
  out "XY Graph 2":cluster{"Y":dbl[], "Y":dbl[]}[](graph)
  out "resolution (ps)":dbl=0.010266666666666667
  in  "file path (dialog if empty)":path=path "C:/Users/User/Data/Jason"
  out "XY Graph":cluster{"Y":dbl[], "Y":dbl[]}[](graph)=[{"Y"=[-0.0006666666666665932, 0.00200000000000015, 0.018000000000000054, 0.028000000000000063, 0.03733333333333348, 0.04666666666666671, 0.05466666666666675, 0.06466666666666676, 0.07600000000000015, 0.08333333333333341, 0.09533333333333338, 0.10533333333333339, 0.11599999999999999, 0.12466666666666681, 0.136, 0.14533333333333343, 0.15666666666666682, 0.16533333333333344, 0.17666666666666683, 0.18600000000000005, 0.19866666666666682, 0.20666666666666667, 0.21866666666666684, 0.22800000000000006, 0.23866666666666667, 0.24866666666666667, 0.2580000000000001, 0.2686666666666667, 0.27866666666666673, 0.2900000000000001, 0.2993333333333335, 0.31133333333333346, 0.31933333333333336, 0.3313333333333335, 0.34066666666666673, 0.35066666666666674, 0.3620000000000001, 0.37133333333333335, 0.3826666666666667, 0.3920000000000001, 0.4033333333333333, 0.41200000000000014, 0.42333333333333334, 0.43333333333333335, 0.44266666666666676, 0.4546666666666668, 0.4640000000000002, 0.4746666666666668, 0.4846666666666668, 0.4946666666666668, 0.5053333333333334, 0.5160000000000001, 0.5253333333333334, 0.5360000000000001, 0.5466666666666669, 0.5573333333333335, 0.5666666666666668, 0.5760000000000001, 0.5873333333333335, 0.5980000000000001, 0.6073333333333335, 0.6186666666666667, 0.6286666666666667, 0.6413333333333334, 0.6473333333333334, 0.6613333333333334, 0.6673333333333334, 0.68, 0.6906666666666668, 0.7000000000000001, 0.7106666666666668, 0.7213333333333334, 0.7313333333333334, 0.7406666666666667, 0.7520000000000001, 0.7653333333333334, 0.7693333333333334, 0.7840000000000001, 0.7926666666666667, 0.8026666666666668, 0.8133333333333335, 0.8240000000000002, 0.8333333333333334, 0.8446666666666668, 0.854, 0.8653333333333335, 0.8746666666666668, 0.8860000000000001, 0.8946666666666668, 0.9046666666666668, 0.9166666666666667, 0.9260000000000002, 0.9366666666666668, 0.9473333333333334, 0.9566666666666668, 0.9666666666666668, 0.9766666666666668, 0.988, 0.9986666666666668, 1.0086666666666668, 1.0193333333333334, 1.0300000000000002, 1.0393333333333334, 1.05, 1.0593333333333335, 1.0693333333333335, 1.082, 1.09, 1.100666666666667, 1.110666666666667, 1.1213333333333335, 1.1300000000000001, 1.1433333333333335, 1.1526666666666667, 1.1620000000000001, 1.1733333333333336, 1.1826666666666668, 1.1933333333333336, 1.2026666666666668, 1.2133333333333336, 1.2246666666666668, 1.2333333333333334, 1.2446666666666668, 1.2560000000000002, 1.2653333333333336, 1.2753333333333337, 1.2846666666666668, 1.2953333333333334, 1.3073333333333335, 1.3160000000000003, 1.3266666666666669, 1.3360000000000003, 1.346666666666667, 1.3573333333333335, 1.366, 1.3773333333333335, 1.3873333333333335, 1.3980000000000001, 1.4073333333333335, 1.4193333333333333, 1.4280000000000002, 1.4393333333333334, 1.4486666666666668, 1.4586666666666668, 1.47, 1.4806666666666668, 1.4906666666666668, 1.5006666666666668, 1.5106666666666668, 1.5206666666666668, 1.5313333333333334, 1.542, 1.552, 1.5626666666666666, 1.5713333333333335, 1.5826666666666667, 1.594, 1.602, 1.614], "Y"=[32.41984123555416, 56.190675667248826, 35.45513007965076, -14.546363436804976, -53.2746629350067, 33.15151342556682, 31.20070509416027, 49.7401093233363, 11.423134889128324, 28.031490458486424, 20.643505634044626, -4.706738819035716, 59.40466080384235, 4.460836803866613, 22.890639415680578, 17.470962316582064, -50.79964016042708, 8.674111354945067, 46.53575222904628, -70.14504456614983, 33.04314192967334, 3.6673844232024253, -29.78911137560148, 21.823258474707615, 85.4069771836224, 29.943057280866476, 76.32657789816616, -72.21137849391803, -24.75458736437011, 59.0960683626989, 82.65539157436451, 34.107076314914146, 112.13402526223084, 37.22024408831476, 62.098983531092884, 11.1888170920106, 74.14197580233657, 65.09711446604354, -0.5398035670290309, 15.006328388539583, 41.77317307116857, 12.4236831631985, 9.698847696267343, -4.352609930183771, 69.82492283560806, -9.268693696581419, 14.791152608141793, -3.8273247727080655, 33.19879530511447, -49.24100284751929, 57.60109759149648, 62.45627883920754, 61.34516956424573, 53.05789894179559, -4.828619151332541, 59.41407052369895, 29.271034587296498, 20.420777436735182, 23.990763756397534, -41.364769358275915, 59.60337397839014, -0.5269478742119205, 91.26688566604003, 36.52413553823507, 30.052650086457426, 48.87383218523819, 63.77806848401411, -28.021408054215897, 93.40912941094564, 133.7356747652147, 87.69748667827571, 1.1427447995563256, 83.44401304159524, 5.360834326982676, 35.545675314518505, 39.621227250206836, -24.366084277159583, -1.1847617966441621, -11.303903769066315, 88.02870587050312, 51.437008628823534, 57.047027698466415, 26.082928240756534, -1.8293049262143164, -12.441164630685849, 21.99683847795584, -25.782237781281463, -18.443166701316414, -46.19286336090777, -39.11106410715824, 53.14819669402617, 32.601411836469815, 3.1317208225006503, 26.60198433342734, 55.46818046140008, -42.35248042159226, 47.45988716438629, 71.73275090456534, 50.06576490346811, -14.97233426564396, -17.188595081284017, 58.572709941401655, 81.01089517974275, 24.629279998872704, 79.37236287781347, 74.75320177011511, 88.47028906574931, -22.857446419032527, -28.261431981046034, -8.174487478135852, 32.284772299381316, -10.89112306361558, 31.288459836075887, -3.822245108599752, 1.7605621583952527, 74.57898876602738, -6.991069685158459, -1.6751518418546942, 17.76745215352156, 38.48501148463486, 37.757350440292264, 2.0426673914727442, -25.74745333314144, 87.0092655317172, 116.77787584830489, -50.22705603898319, -43.67426919819431, 27.61319181234582, 1.1413902148232893, 5.0480921880360015, 38.04928083829648, -48.03521291204768, -13.738891906939843, -27.580773596761563, 28.1376277390964, 43.82817011530041, 21.409668047445678, 33.88034581504324, 19.2108222319626, 48.21766777893829, 82.44511994885315, 14.198410539476907, 23.637294213136386, -3.672969592776669, 61.26264633523048, 17.092705358964626, -15.728798247011586, 11.88008030183984, 92.86970867286641, 7.599122147214187, 26.10824115003115, 3.6544583251546783, 11.738134408612277, -25.55539228949919, 78.14378420471841, 30.614099728542804, 64.83056368356671, 28.700204296906282, 19.203309222293967]}, {"Y"=[-0.0006666666666665932, 0.00200000000000015, 0.018000000000000054, 0.028000000000000063, 0.03733333333333348, 0.04666666666666671, 0.05466666666666675, 0.06466666666666676, 0.07600000000000015, 0.08333333333333341, 0.09533333333333338, 0.10533333333333339, 0.11599999999999999, 0.12466666666666681, 0.136, 0.14533333333333343, 0.15666666666666682, 0.16533333333333344, 0.17666666666666683, 0.18600000000000005, 0.19866666666666682, 0.20666666666666667, 0.21866666666666684, 0.22800000000000006, 0.23866666666666667, 0.24866666666666667, 0.2580000000000001, 0.2686666666666667, 0.27866666666666673, 0.2900000000000001, 0.2993333333333335, 0.31133333333333346, 0.31933333333333336, 0.3313333333333335, 0.34066666666666673, 0.35066666666666674, 0.3620000000000001, 0.37133333333333335, 0.3826666666666667, 0.3920000000000001, 0.4033333333333333, 0.41200000000000014, 0.42333333333333334, 0.43333333333333335, 0.44266666666666676, 0.4546666666666668, 0.4640000000000002, 0.4746666666666668, 0.4846666666666668, 0.4946666666666668, 0.5053333333333334, 0.5160000000000001, 0.5253333333333334, 0.5360000000000001, 0.5466666666666669, 0.5573333333333335, 0.5666666666666668, 0.5760000000000001, 0.5873333333333335, 0.5980000000000001, 0.6073333333333335, 0.6186666666666667, 0.6286666666666667, 0.6413333333333334, 0.6473333333333334, 0.6613333333333334, 0.6673333333333334, 0.68, 0.6906666666666668, 0.7000000000000001, 0.7106666666666668, 0.7213333333333334, 0.7313333333333334, 0.7406666666666667, 0.7520000000000001, 0.7653333333333334, 0.7693333333333334, 0.7840000000000001, 0.7926666666666667, 0.8026666666666668, 0.8133333333333335, 0.8240000000000002, 0.8333333333333334, 0.8446666666666668, 0.854, 0.8653333333333335, 0.8746666666666668, 0.8860000000000001, 0.8946666666666668, 0.9046666666666668, 0.9166666666666667, 0.9260000000000002, 0.9366666666666668, 0.9473333333333334, 0.9566666666666668, 0.9666666666666668, 0.9766666666666668, 0.988, 0.9986666666666668, 1.0086666666666668, 1.0193333333333334, 1.0300000000000002, 1.0393333333333334, 1.05, 1.0593333333333335, 1.0693333333333335, 1.082, 1.09, 1.100666666666667, 1.110666666666667, 1.1213333333333335, 1.1300000000000001, 1.1433333333333335, 1.1526666666666667, 1.1620000000000001, 1.1733333333333336, 1.1826666666666668, 1.1933333333333336, 1.2026666666666668, 1.2133333333333336, 1.2246666666666668, 1.2333333333333334, 1.2446666666666668, 1.2560000000000002, 1.2653333333333336, 1.2753333333333337, 1.2846666666666668, 1.2953333333333334, 1.3073333333333335, 1.3160000000000003, 1.3266666666666669, 1.3360000000000003, 1.346666666666667, 1.3573333333333335, 1.366, 1.3773333333333335, 1.3873333333333335, 1.3980000000000001, 1.4073333333333335, 1.4193333333333333, 1.4280000000000002, 1.4393333333333334, 1.4486666666666668, 1.4586666666666668, 1.47, 1.4806666666666668, 1.4906666666666668, 1.5006666666666668, 1.5106666666666668, 1.5206666666666668, 1.5313333333333334, 1.542, 1.552, 1.5626666666666666, 1.5713333333333335, 1.5826666666666667, 1.594, 1.602, 1.614], "Y"=[-11.362481873506388, 37.3354737008185, -31.03715607855192, -45.856294329988536, 10.818389165135667, 6.860735219327868, -3.9174136446856256, 9.845371015991795, -18.47331956587059, -10.059251131299137, -13.34750386396259, -19.46794923371829, -2.4503332648140166, 68.95768499079372, 58.71849975102165, 10.093737436024533, -73.7300075250331, -22.489769957362746, 39.156132358899356, 59.46146109199717, -74.88763163612194, 14.52469919831793, 9.75107846470099, -6.218397807428495, 48.62896597278261, 96.07229554146889, 23.45708982646522, -30.324470036758562, 30.491183333915593, -45.199853049229205, -6.553053568462531, 25.730955349906807, 44.215235866829495, -49.450359617302325, 24.201208774762353, 9.123568370548165, -15.735833872414606, -1.3225130971051335, -13.355329150572143, 48.88968415745785, -25.315476224995933, 16.16402511297832, 43.47381232974995, -30.982801318149807, 32.208308190988745, 43.134231280637664, 8.916200120940044, 22.04450482671136, 26.031374893208667, -11.294838421393067, 23.61425382877718, -18.851939541926175, -40.483674493562596, 62.51156942005455, -21.56795443559065, 57.01123138109253, -108.40564097923757, -27.31666058031033, -30.70213585384309, -42.53864237690272, 50.90952931941057, -38.49410826614776, 71.39267339109298, 40.07683898022668, -0.09411896982421375, 77.62129886482327, -1.8244852175589408, 21.80583893940247, 104.1991017748611, 14.048658707627816, -13.318276474398303, 67.53927402899974, -24.14901754885396, -23.72667584814341, -43.87187806914632, 37.04887648989405, -17.334175480085694, -24.166929901648373, 14.481497085623458, -61.76882887171625, -22.999516053298848, -69.89240347692099, -3.434820058648217, 21.867017329985483, -26.999665202291936, -3.3632444004583686, -37.082195733307, 55.610461403368234, -1.4819186333156082, 34.02327779472803, 22.531615675545677, -28.90121881843004, 43.01814742201887, 58.59459542126888, 50.19644658968815, 32.93664905062978, 11.572233832681352, 29.268992467647593, -68.11713435384135, -0.07265062793137389, -12.200447610358898, 35.64183609426206, 40.30361852929323, 47.03447847917832, 39.398316468108064, 41.018364335251704, -17.13995341893896, -32.37090470076058, -34.94978623675682, -45.17366696234411, 0.30271022103302236, -68.56838773985677, 7.432436998017307, 71.1254517750013, 87.99586264298617, 2.894798581538396, -36.076591445698604, -5.2223421161967805, -36.165456434301845, 24.525650511660892, 46.036969404909506, -7.533168182109867, 32.78649244400704, 11.005442567356276, 21.174863719219452, 41.16810975117491, -45.86218241797435, 61.66373621472306, -38.56019580462675, -69.8333514181696, 41.16402009876934, 38.18516378007271, -29.948083774579572, -14.680366944662037, -24.43495605347761, 85.01985743317503, -9.052094655083165, -11.680939261949973, -28.22775071188835, 20.0423001712938, -29.472884296354266, -16.001424858382574, -12.144112442994896, 21.41755956567104, -46.02223005960271, -16.20555830897209, -26.994365350506758, -100.31017928213917, 49.489156097079196, 6.7363442754774425, -47.38668542381265, 13.943766459811663, 25.017556280616738, -38.09182804955434, 28.051215319657413, 41.26025649512321, -19.047343605681906, 44.781778813621656, 66.17464305614624]}]
  out "Count":dbl=1434.0
  out "sum":dbl(graph)=6546.3048000460785
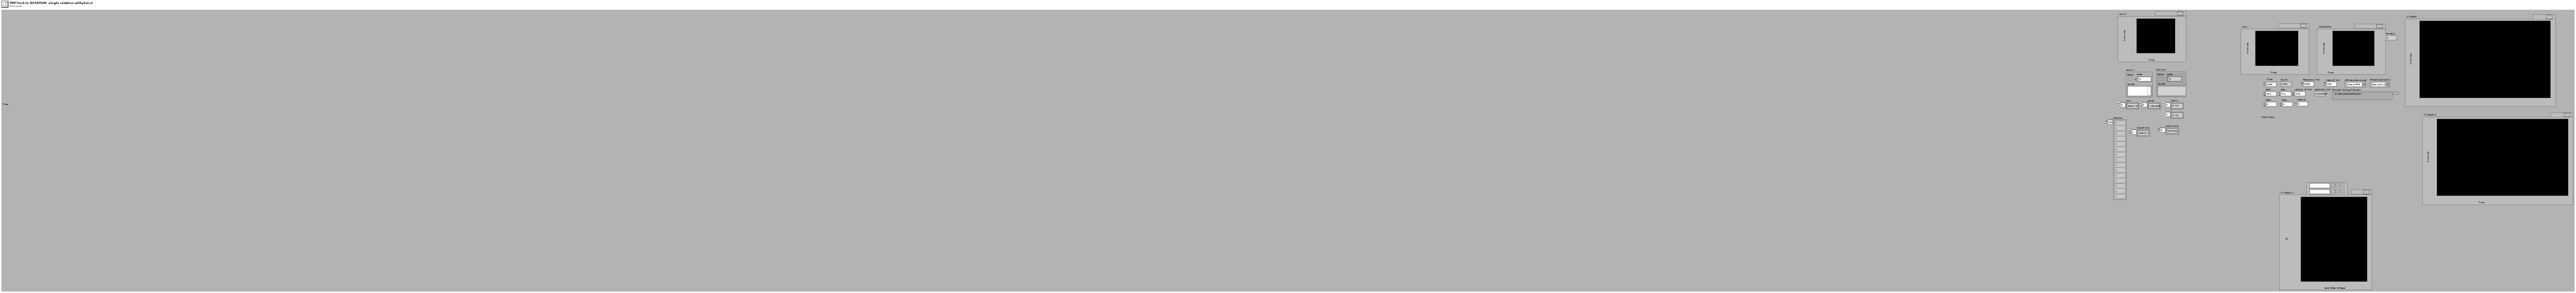
[diagram p1: front panel]
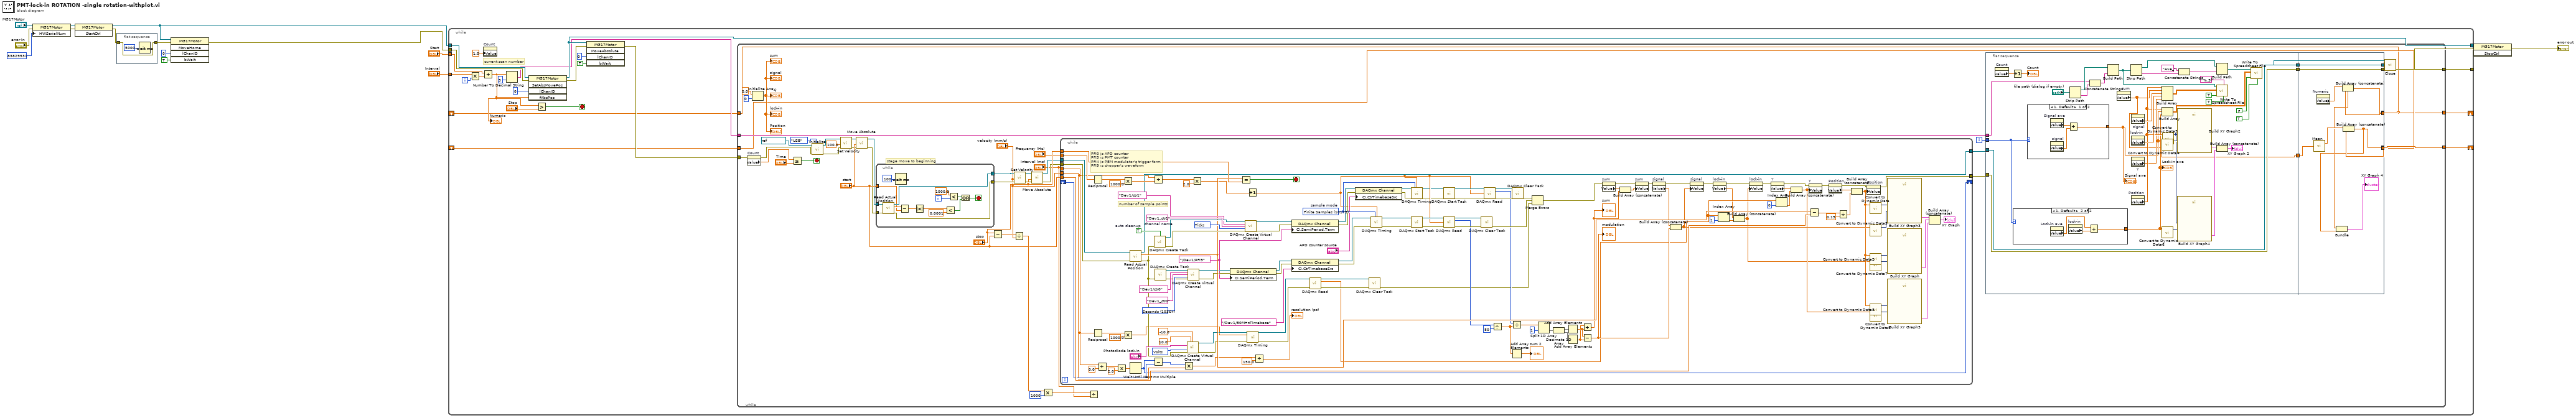
[diagram p0: block diagram]
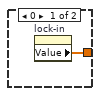
[diagram p2: hidden frame]
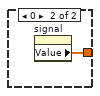
[diagram p3: hidden frame]
diagram:
  n1 = property class="MG17Motor"(reference="MG17Motor", error in="error in", "HWSerialNum"=83829531) -> (reference out=w12:refnum<k7>, error out=w11:errorcluster)
  n2 = invoke class="MG17Motor" method="StartCtrl"(reference=w12, error in=w11) -> (reference out=w7:refnum<k7>, error out=w6:errorcluster)  [unwired: 1 in, 1 out]
  n3 = flat-sequence {
    tunnel: w6 -> [w18]
    tunnel: [w18] -> w5
    frame #0 {
      n4 = Wait (ms)(milliseconds to wait=u32 5000) -> ()  [unwired: 1 out]
    }
  }
  n5 = invoke class="MG17Motor" method="MoveHome"(reference=w7, error in=w5, "lChanID"=0, "bWait"=TRUE) -> (error out=w1:errorcluster)  [unwired: 1 in, 4 out]
  n6 = while {
    tunnel: "Start" -> [w40]
    tunnel: "Interval" -> [w39]
    tunnel: w1 -> [w35]
    tunnel: w7 -> [w34]
    tunnel: [w32] -> w9
    tunnel: [w31] -> w8
    shift-right: [w23] -> _
    shift-left: _ -> [w22]
    shift-right: [w20] -> _
    shift-left: _ -> [w19]
    i -> [w38]
    stop <- w36 stop-if-true
    # "current scan number"
    n7 = Multiply(x=w39, y=w38) -> (x*y=w37:dbl)
    n8 = Add(x=w40, y=w37) -> (x+y=w21:dbl)
    "Numeric" <- w21
    n9 = property on="Count" class="DigNum (strict)"("Value"=1.0 ("Count")) -> ()  [unwired: 2 in, 2 out]
    n10 = Number To Decimal String(number=w21, width (-)=i16 3) -> (decimal integer string=w29:string)
    n11 = invoke class="MG17Motor" method="SetAbsMovePos"(reference=w34, error in=w35, "lChanID"=0, "fAbsPos"=w21) -> (reference out=w31:refnum<k7>, error out=w33:errorcluster)  [unwired: 1 in, 3 out]
    n12 = Greater?(x=w21, y="Stop") -> (0:w36:bool)
    n13 = invoke class="MG17Motor" method="MoveAbsolute"(reference=w31, error in=w33, "lChanID"=0, "bWait"=TRUE) -> (error out=w24:errorcluster)  [unwired: 1 in, 4 out]
    n14 = while {
      tunnel: w24 -> [w64]
      tunnel: [w52] -> w32
      tunnel: w29 -> [w49]
      tunnel: [w45] -> w23
      tunnel: w22 -> [w44]
      tunnel: [w43] -> w20
      tunnel: w19 -> [w42]
      i -> [w61]
      stop <- w67 stop-if-true
      # "stage move to beginning"
      n15 = property on="Count" class="DigNum (strict)"(error in=w64) -> (error out=w63:errorcluster, "Value"=w62:dbl)  [unwired: 1 in, 1 out]
      n16 = Initialize Array(0.0 ("element"), 0 ("dimension size")) -> (→"sum" →"signal" →"Position" →"lock-in" →"Y":dbl[])
      n17 = Greater Or Equal?(x=w62, y="Time") -> (x >= y?=w67:bool)
      n18 = call <userlib>:"Initialize.vi"("VISA resource name"=refnum<visa-resource-name> "COM12", "error in (no error)"=w63, "Serial Link (RS232)"=enum16{"RS232", "USB"}."USB") -> ("VISA resource name out"=w55:refnum<visa-resource-name>, "error out"=w56:errorcluster)  [unwired: 6 in]
      n19 = call <userlib>:"Set Velocity.vi"("error in (no error)"=w56, "Velocity (units/s)"=100.0 ("value (0)"), "VISA resource name"=w55) -> ("error out"=w59:errorcluster, "VISA resource name out"=w60:refnum<visa-resource-name>)  [unwired: 3 in]
      n20 = call <userlib>:"Move Absolute.vi"("error in (no error)"=w59, "Position (0 units)"="start", "VISA resource name"=w60) -> ("error out"=w57:errorcluster, "VISA resource name out"=w58:refnum<visa-resource-name>)  [unwired: 3 in]
      n21 = while {
        tunnel: "start" -> [w89]
        tunnel: w58 -> [w101]
        tunnel: w57 -> [w100]
        tunnel: [w95] -> w78
        tunnel: [w96] -> w80
        i -> [w98]
        stop <- w97 stop-if-true
        n22 = call <userlib>:"Read Actual Position.vi"("error in (no error)"=w100, "VISA resource name"=w101) -> ("error out"=w95:errorcluster, "Position (units)"=w90:dbl, "VISA resource name out"=w96:refnum<visa-resource-name>)  [unwired: 3 in]
        n23 = Wait (ms)(milliseconds to wait=u32 100) -> ()  [unwired: 1 out]
        n24 = Subtract(x=w90, y=w89) -> (x-y=w93:dbl)
        n25 = Absolute Value(x=w93) -> (abs(x)=w92:dbl)
        n26 = Less?(x=w92, y=0.0001) -> (x < y?=w88:bool)
        n27 = Less?(x=1000.0, y=w98) -> (x < y?=w94:bool)
        n28 = Or(x=w94, y=w88) -> (x .or. y?=w97:bool)
      }
      n29 = Subtract(x="stop", y="start") -> (x-y=w87:dbl)
      n30 = Divide(x=w87, y="velocity (mm/s)") -> (x/y=w85:dbl)
      n31 = call <userlib>:"Set Velocity.vi"("error in (no error)"=w78, "Velocity (units/s)"="velocity (mm/s)", "VISA resource name"=w80) -> ("error out"=w77:errorcluster, "VISA resource name out"=w79:refnum<visa-resource-name>)  [unwired: 3 in]
      n32 = call <userlib>:"Move Absolute.vi"("error in (no error)"=w77, "Position (0 units)"="stop", "VISA resource name"=w79) -> ("error out"=w74:errorcluster, "VISA resource name out"=w75:refnum<visa-resource-name>)  [unwired: 3 in]
      n33 = Multiply(x=w85, y=1000) -> (x*y=w84:dbl)
      n34 = while {
        tunnel: "Frequency (Hz)" -> [w276]
        tunnel: "stop" -> [w275]
        tunnel: "start" -> [w273]
        tunnel: w75 -> [w269]
        tunnel: w74 -> [w268]
        tunnel: [w211] -> w68
        tunnel: [w266] -> w69
        shift-right: [w235] -> _
        shift-left: _ -> [w241]
        tunnel: "velocity (mm/s)" -> [w236]
        tunnel: "Interval (ms)" -> [w180]
        stop <- w274 stop-if-true
        w164 = 10348 items=["Volts"=10348, "From Custom Scale"=10065] ("units")
        w204 = tag "/Dev1/PFI9" ("CI.SemiPeriod.Term")
        w261 = 10364 items=["Seconds"=10364, "Ticks"=10304, "From Custom Scale"=10065] ("units")
        w290 = 10304 items=["Seconds"=10364, "Ticks"=10304, "From Custom Scale"=10065] ("units")
        w257 = 10178 items=["Finite Samples"=10178, "Continuous Samples"=10123, "Hardware Timed Single Point"=12522]  # sample mode
        w291 = "Dev1_ctr1"  # channel name
        w292 = TRUE  # auto cleanup
        # "number of sample points"
        # "PFI0 is APD counter\nPFI3 is PMT counter\nPFI4 is PEM modulator's trigger form\nPFI9 is chopper's waveform"
        n35 = Reciprocal(x=w276) -> (1/x=w280:dbl)
        n36 = Reciprocal(x=w180) -> (1/x=w181:dbl)
        n37 = Add(x=w180, y=0.0) -> (x+y=w233:dbl)
        n38 = Multiply(x=w233, y=2.0) -> (x*y=w209:dbl)
        n39 = Multiply(x=w280, y=1000.0) -> (x*y=w278:dbl)
        n40 = Multiply(x=w181, y=1000.0) -> (x*y=w174:dbl)
        n41 = call <userlib>:"Read Actual Position.vi"("error in (no error)"=w268, "VISA resource name"=w269) -> ("error out"=w177:errorcluster, "Position (units)"=w270:dbl, "VISA resource name out"=w266:refnum<visa-resource-name>)  [unwired: 3 in]
        n42 = Wait Until Next ms Multiple(millisecond multiple=w209) -> (millisecond timer value=w235:u32)
        n43 = Divide(x=w180, y=w278) -> (x/y=w242:dbl)
        n44 = Subtract(x=w235, y=w241) -> (x-y=w237:u32)
        n45 = call <vilib>:"DAQmx Create Task.vi"("auto cleanup"=w292, "error in"=w177) -> ("task out"=w289:refnum<k21>, "error out"=w288:errorcluster)  [unwired: 12 in]
        n46 = call <vilib>:"DAQmx Create Task.vi"("error in"=w177) -> ("task out"=w265:refnum<k21>, "error out"=w260:errorcluster)  [unwired: 13 in]
        n47 = Multiply(x=w237, y=w236) -> (x*y=w239:dbl)
        n48 = call-poly <vilib>:"DAQmx Create Virtual Channel.vi"("maximum value"=10.0, "minimum value"=-10.0, "physical channels"="Photodiode lock-in", "units"=w164, "error in"=w177) -> ("task out"=w186:refnum<k21>, "error out"=w184:errorcluster)  [unwired: 9 in]
        n49 = call-poly <vilib>:"DAQmx Create Virtual Channel.vi"("task in"=w265, "counter"=tag "Dev1/ctr0", "name to assign"="Dev1_ctr0", "units"=w261, "error in"=w260) -> ("task out"=w250:refnum<k21>, "error out"=w249:errorcluster)  [unwired: 9 in]
        n50 = Multiply(x=w242, y=2.0) -> (x*y=w190:dbl)
        n51 = property class="DAQmx Channel"(reference=w250, error in=w249, "CI.SemiPeriod.Term"=w204) -> (reference out=w248:refnum<k21>, error out=w247:errorcluster)
        n52 = Equal?(x=w270, y=w275) -> (x = y?=w274:bool)
        n53 = call-poly <vilib>:"DAQmx Create Virtual Channel.vi"("task in"=w289, "counter"=tag "Dev1/ctr1", "name to assign"=w291, "units"=w290, "error in"=w288) -> ("task out"=w230:refnum<k21>, "error out"=w228:errorcluster)  [unwired: 9 in]
        n54 = Increment(x=w190) -> (x+1=w226:dbl)
        n55 = call-poly <vilib>:"DAQmx Timing.vi"("task/channels in"=w186, "rate"=w174, "error in"=w184) -> ("task out"=w185:refnum<k21>, "error out"=w183:errorcluster)  [unwired: 11 in]
        n56 = Divide(x=w239, y=150.0) -> (x/y=→"resolution (ps)":dbl)
        n57 = property class="DAQmx Channel"(reference=w230, error in=w228, "CI.SemiPeriod.Term"=w204) -> (reference out=w229:refnum<k21>, error out=w227:errorcluster)
        n58 = property class="DAQmx Channel"(reference=w248, error in=w247, "CI.CtrTimebaseSrc"=tag "/Dev1/80MHzTimebase") -> (reference out=w259:refnum<k21>, error out=w258:errorcluster)
        n59 = call-poly <vilib>:"DAQmx Read.vi"("task/channels in"=w185, "error in"=w183) -> ("task out"=w198:refnum<k21>, "data"=w160:dbl[], "error out"=w197:errorcluster)  [unwired: 11 in]
        n60 = property class="DAQmx Channel"(reference=w229, error in=w227, "CI.CtrTimebaseSrc"="APD counter source") -> (reference out=w286:refnum<k21>, error out=w285:errorcluster)
        n61 = call <vilib>:"DAQmx Clear Task.vi"("task in"=w198, "error in"=w197) -> ("error out"=w187:errorcluster)  [unwired: 13 in]
        n62 = call-poly <vilib>:"DAQmx Timing.vi"("task/channels in"=w259, "sample mode"=w257, "samples per channel"=w226, "error in"=w258) -> ("task out"=w206:refnum<k21>, "error out"=w207:errorcluster)  [unwired: 10 in]
        n63 = call-poly <vilib>:"DAQmx Timing.vi"("task/channels in"=w286, "sample mode"=w257, "samples per channel"=w226, "error in"=w285) -> ("task out"=w205:refnum<k21>, "error out"=w208:errorcluster)  [unwired: 10 in]
        n64 = call <vilib>:"DAQmx Start Task.vi"("task/channels in"=w206, "error in"=w207) -> ("task out"=w256:refnum<k21>, "error out"=w255:errorcluster)  [unwired: 12 in]
        n65 = call <vilib>:"DAQmx Start Task.vi"("task/channels in"=w205, "error in"=w208) -> ("task out"=w284:refnum<k21>, "error out"=w283:errorcluster)  [unwired: 12 in]
        n66 = call-poly <vilib>:"DAQmx Read.vi"("task/channels in"=w256, "number of samples per channel"=w226, "error in"=w255) -> ("task out"=w254:refnum<k21>, "data"=w244:u32[], "error out"=w253:errorcluster)  [unwired: 10 in]
        n67 = call <vilib>:"DAQmx Clear Task.vi"("task in"=w254, "error in"=w253) -> ("error out"=w252:errorcluster)  [unwired: 13 in]
        n68 = call-poly <vilib>:"DAQmx Read.vi"("task/channels in"=w284, "number of samples per channel"=w226, "error in"=w283) -> ("task out"=w282:refnum<k21>, "data"=w251:u32[], "error out"=w281:errorcluster)  [unwired: 10 in]
        n69 = Divide(x=w244, y=80) -> (x/y=w245:dbl[])
        n70 = Divide(x=w251, y=w245) -> (x/y=w223:dbl[])
        n71 = Add Array Elements(numeric array=w245) -> (sum=→"sum 2":dbl)
        n72 = call <vilib>:"DAQmx Clear Task.vi"("task in"=w282, "error in"=w281) -> ("error out"=w267:errorcluster)  [unwired: 13 in]
        n73 = Merge Errors(w267, w252, w187) -> (w188:errorcluster)
        n74 = Split 1D Array(array=w223, index=1 ("length")) -> (second subarray=w225:dbl[])  [unwired: 1 out]
        n75 = Decimate 1D Array(w225) -> (w203:dbl[], w202:dbl[])
        n76 = Add Array Elements(numeric array=w203) -> (sum=w201:dbl)
        n77 = Add Array Elements(numeric array=w202) -> (sum=w200:dbl)
        n78 = Add(x=w200, y=w201) -> (x+y=w219:dbl)
        "sum" <- w219
        n79 = Subtract(x=w201, y=w200) -> (x-y=w216:dbl)
        "modulation" <- w216
        n80 = property on="sum" class="Arr (strict)"(error in=w188) -> (error out=w215:errorcluster, "Value"=w220:cdb[])  [unwired: 1 in, 1 out]
        n81 = Build Array (concatenate)(w220, w219) -> (w218:cdb[])
        n82 = property on="sum" class="Arr (strict)"(error in=w215, "Value"=w218) -> (error out=w214:errorcluster)  [unwired: 1 in, 1 out]
        n83 = property on="signal" class="Arr (strict)"(error in=w214) -> (error out=w193:errorcluster, "Value"=w217:cdb[])  [unwired: 1 in, 1 out]
        n84 = Build Array (concatenate)(w217, w216) -> (w194:cdb[])
        n85 = property on="signal" class="Arr (strict)"(error in=w193, "Value"=w194) -> (error out=w192:errorcluster)  [unwired: 1 in, 1 out]
        n86 = property on="lock-in" class="Arr (strict)"(error in=w192) -> (error out=w191:errorcluster, "Value"=w158:cdb[])  [unwired: 1 in, 1 out]
        n87 = Index Array(array=w160, index=1) -> (element=w159:dbl)
        n88 = Build Array (concatenate)(w158, w159) -> (w157:cdb[])
        n89 = property on="lock-in" class="Arr (strict)"(error in=w191, "Value"=w157) -> (error out=w167:errorcluster)  [unwired: 1 in, 1 out]
        n90 = property on="Y" class="Arr (strict)"(error in=w167) -> (error out=w175:errorcluster, "Value"=w176:cdb[])  [unwired: 1 in, 1 out]
        n91 = Index Array(array=w160, index=0) -> (element=w161:dbl)
        n92 = Build Array (concatenate)(w176, w161) -> (w170:cdb[])
        n93 = property on="Y" class="Arr (strict)"(error in=w175, "Value"=w170) -> (error out=w166:errorcluster)  [unwired: 1 in, 1 out]
        n94 = Subtract(x=w270, y=w273) -> (x-y=w272:dbl)
        n95 = property on="Position" class="Arr (strict)"(error in=w166) -> (error out=w212:errorcluster, "Value"=w213:dbl[])  [unwired: 1 in, 1 out]
        n96 = Divide(x=w272, y=0.15) -> (x/y=w210:dbl)
        n97 = Build Array (concatenate)(w213, w210) -> (w172:dbl[])
        n98 = property on="Position" class="Arr (strict)"(error in=w212, "Value"=w172) -> (error out=w211:errorcluster)  [unwired: 1 in, 1 out]
        n99 = call "Convert to Dynamic Data"("Array"=w172) -> ("Dynamic Data Type"=w222:dynamicdata)  [unwired: 3 in]
        n100 = call "Convert to Dynamic Data5"("Array"=w194) -> ("Dynamic Data Type"=w221:dynamicdata)  [unwired: 3 in]
        n101 = call "Convert to Dynamic Data2"("Array"=w172) -> ("Dynamic Data Type"=w195:dynamicdata)  [unwired: 3 in]
        n102 = call "Convert to Dynamic Data7"("Array"=w157) -> ("Dynamic Data Type"=w189:dynamicdata)  [unwired: 3 in]
        n103 = call "Convert to Dynamic Data8"("Array"=w172) -> ("Dynamic Data Type"=w173:dynamicdata)  [unwired: 3 in]
        n104 = call "Convert to Dynamic Data9"("Array"=w170) -> ("Dynamic Data Type"=w171:dynamicdata)  [unwired: 3 in]
        n105 = call "Build XY Graph3"("Y Input"=w221, "X Input"=w222) -> ("XY Graph"=w168:cluster{"Y":dbl[], "Y":dbl[]}[])  [unwired: 3 in, 6 out]
        n106 = call "Build XY Graph"("Y Input"=w189, "X Input"=w195) -> ("XY Graph"=w196:cluster{"Y":dbl[], "Y":dbl[]}[])  [unwired: 3 in, 6 out]
        n107 = call "Build XY Graph5"("Y Input"=w171, "X Input"=w173) -> ("XY Graph"=w169:cluster{"Y":dbl[], "Y":dbl[]}[])  [unwired: 3 in, 6 out]
        n108 = Build Array (concatenate)(w168, w196, w169) -> (→"XY Graph":cluster{"Y":dbl[], "Y":dbl[]}[])
      }
      n109 = Divide(x=w84, y="Interval (ms)") -> ()  [unwired: 1 out]
      n110 = flat-sequence {
        tunnel: w69 -> [w129]
        tunnel: w68 -> [w128]
        tunnel: w61 -> [w126]
        tunnel: w49 -> [w106]
        tunnel: [w129] -> w48
        tunnel: [w128] -> w47
        tunnel: [w103] -> w46
        tunnel: [w155] -> w54
        tunnel: [w156] -> w53
        tunnel: w48 -> [w156]
        tunnel: w47 -> [w155]
        tunnel: w46 -> [w154]
        tunnel: [w151] -> w45
        tunnel: w44 -> [w152]
        tunnel: [w147] -> w43
        tunnel: w42 -> [w148]
        frame #0 {
          n111 = property on="Count" class="DigNum (strict)"() -> ("Value"=w131:dbl)  [unwired: 2 in, 2 out]
          n112 = Increment(x=w131) -> (x+1=→"Count":dbl)
          n113 = case shown="1, Default" w126 {
            tunnel: [w139 w141] -> w113
            frame 0 {
              n114 = property on="lock-in" class="Arr (strict)"() -> ("Value"=w139:cdb[])  [unwired: 2 in, 2 out]
            }
            frame 1, Default {
              n115 = property on="Lock-in ave" class="Arr (strict)"() -> ("Value"=w142:cdb[])  [unwired: 2 in, 2 out]
              n116 = property on="lock-in" class="Arr (strict)"() -> ("Value"=w140:cdb[])  [unwired: 2 in, 2 out]
              n117 = Add(x=w142, y=w140) -> (x+y=w141:cdb[])
            }
          }
          "Lock-in ave" <- w113
          n118 = case shown="1, Default" w126 {
            tunnel: [w145 w146] -> w104
            frame 1, Default {
              n119 = property on="Signal ave" class="Arr (strict)"() -> ("Value"=w144:cdb[])  [unwired: 2 in, 2 out]
              n120 = property on="signal" class="Arr (strict)"() -> ("Value"=w143:cdb[])  [unwired: 2 in, 2 out]
              n121 = Add(x=w144, y=w143) -> (x+y=w145:cdb[])
            }
            frame 0 {
              n122 = property on="signal" class="Arr (strict)"() -> ("Value"=w146:cdb[])  [unwired: 2 in, 2 out]
            }
          }
          "Signal ave" <- w104
          n123 = Strip Path(path="file path (dialog if empty)") -> (stripped path=w110:path, name=w105:string)
          n124 = Concatenate Strings(w106, w105) -> (w109:string)
          n125 = Build Path(base path=w110, name or relative path=w109) -> (appended path=w107:path)
          n126 = property on="sum" class="Arr (strict)"() -> ("Value"=w103:cdb[])  [unwired: 2 in, 2 out]
          n127 = Strip Path(path=w107) -> (stripped path=w119:path, name=w117:string)
          n128 = property on="signal" class="Arr (strict)"() -> ("Value"=w125:cdb[])  [unwired: 2 in, 2 out]
          n129 = property on="lock-in" class="Arr (strict)"() -> ("Value"=w124:cdb[])  [unwired: 2 in, 2 out]
          n130 = property on="Y" class="Arr (strict)"() -> ("Value"=w112:cdb[])  [unwired: 2 in, 2 out]
          n131 = property on="Position" class="Arr (strict)"() -> ("Value"=w114:dbl[])  [unwired: 2 in, 2 out]
          n132 = Build Array(w114, w103, w125, w124, w112) -> (w123:cdb[][])
          n133 = Build Array(w114, w104, w113) -> (w111:cdb[][])
          n134 = call "Convert to Dynamic Data4"("Array"=w104) -> ("Dynamic Data Type"=w134:dynamicdata)  [unwired: 3 in]
          n135 = call "Convert to Dynamic Data6"("Array"=w113) -> ("Dynamic Data Type"=w135:dynamicdata)  [unwired: 3 in]
          n136 = call "Convert to Dynamic Data3"("Array"=w114) -> ("Dynamic Data Type"=w127:dynamicdata)  [unwired: 3 in]
          n137 = call "Build XY Graph2"("Y Input"=w134, "X Input"=w127) -> ("XY Graph"=w136:cluster{"Y":dbl[], "Y":dbl[]}[])  [unwired: 3 in, 6 out]
          n138 = call "Build XY Graph4"("Y Input"=w135, "X Input"=w127) -> ("XY Graph"=w137:cluster{"Y":dbl[], "Y":dbl[]}[])  [unwired: 3 in, 6 out]
          n139 = Concatenate Strings("Ave_" ("name or relative path"), w117) -> (w118:string)
          n140 = Build Path(base path=w119, name or relative path=w118) -> (appended path=w115:path)
          n141 = call-poly <vilib>:"Write To Spreadsheet File.vi"("transpose? (no:F)"=TRUE, "format (%.3f)"="%.3f", "append to file? (new file:F)"=TRUE, "2D data"=w123, "file path (dialog if empty)"=w107) -> ()  [unwired: 3 in, 1 out]
          n142 = Build Array (concatenate)(w136, w137) -> (→"XY Graph 2":cluster{"Y":dbl[], "Y":dbl[]}[])
          n143 = call-poly <vilib>:"Write To Spreadsheet File.vi"("transpose? (no:F)"=TRUE, "append to file? (new file:F)"=FALSE, "2D data"=w111, "file path (dialog if empty)"=w115) -> ()  [unwired: 4 in, 1 out]
        }
        frame #1 {
          n144 = call <vilib>:"Mean.vi"("X"=w154) -> ("mean"=w153:dbl)  [unwired: 1 out]
          n145 = property on="Numeric" class="DigNum (strict)"() -> ("Value"=w149:dbl)  [unwired: 2 in, 2 out]
          n146 = Build Array (concatenate)(w149, w148) -> (w147:dbl[])
          n147 = Build Array (concatenate)(w153, w152) -> (w151:dbl[])
          n148 = Bundle(w147, w151) -> (→"XY Graph 4":cluster{dbl[], dbl[]})  [unwired: 1 in]
        }
      }
      n149 = call <userlib>:"Close.vi"("error in (no error)"=w54, "VISA resource name"=w53) -> ("error out"=w52:errorcluster)  [unwired: 9 in]
    }
  }
  n150 = invoke class="MG17Motor" method="StopCtrl"(reference=w8, error in=w9) -> (error out=→"error out":errorcluster)  [unwired: 1 in, 2 out]
